vi "Destructor.vi"(8 "error in (no error)":errorcluster, 11 "WindowFrame in":refnum<class "WindowFrame.lvclass">) -> (0 "error out":errorcluster)   [LabVIEW 2021, in "WindowFrame.lvlib" / "WindowFrame.lvclass"]
uses:
  WindowFrame.lvclass
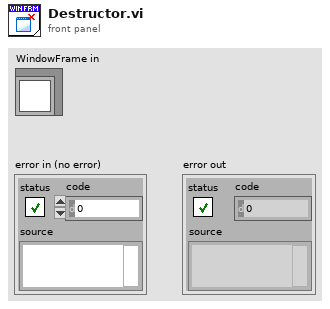
[diagram p1: front panel]
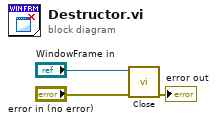
[diagram p0: block diagram]
diagram:
  n1 = call "Close.vi"("error in (no error)"="error in (no error)", "WindowFrame in"="WindowFrame in") -> ("error out"=→"error out":errorcluster)  [unwired: 9 in]
